vi "U16ToByte.vi"(11 "数值":u16) -> (2 "高8位":u8, 3 "低8位":u8)   [LabVIEW 2018]
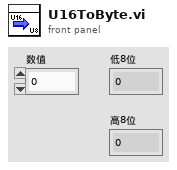
[diagram p1: front panel]
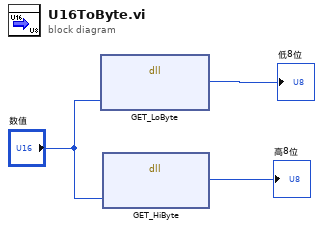
[diagram p0: block diagram]
diagram:
  n1 = dll-call lib="PTH2tabs CUsersadminDesktop'完善2020版本zlgcan_labview_20220510zlgcan_demo_CANET_UDPbinzlgcan_wrap.dll" fn="GET_LoByte"("U16(IN)"="数值") -> ("返回类型"=→"低8位":u8)  [unwired: 4 in, 2 out]
  n2 = dll-call lib="PTH2tabs CUsersadminDesktop'完善2020版本zlgcan_labview_20220510zlgcan_demo_CANET_UDPbinzlgcan_wrap.dll" fn="GET_HiByte"("U16(IN)"="数值") -> ("返回类型"=→"高8位":u8)  [unwired: 4 in, 2 out]
